vi "_visitCompoundGraphic.vi"(8 "error in (no error)":errorcluster, 10 "CompoundShape":refnum<class "CompoundShape.lvclass">, 11 "XMLExportVisitor in":refnum<class "XMLExportVisitor.lvclass">) -> (0 "error out":errorcluster, 2 "String":string, 3 "XMLExportVisitor out":refnum<class "XMLExportVisitor.lvclass">)   [LabVIEW 2018, in "XMLExportVisitor.lvclass"]
uses:
  XMLExportVisitor.lvclass
  C:/Users/fflores/Documents/LabVIEW-Open-Projects/LabIVEW OOP Design Patterns/Visitor Pattern/Visitor Class/Visitor.lvclass
  CompoundShape Class/CompoundShape.lvclass
  CompoundShape Class/CompoundShape.lvclass/CompoundShape.ctl
  Shape Class/Shape.lvclass
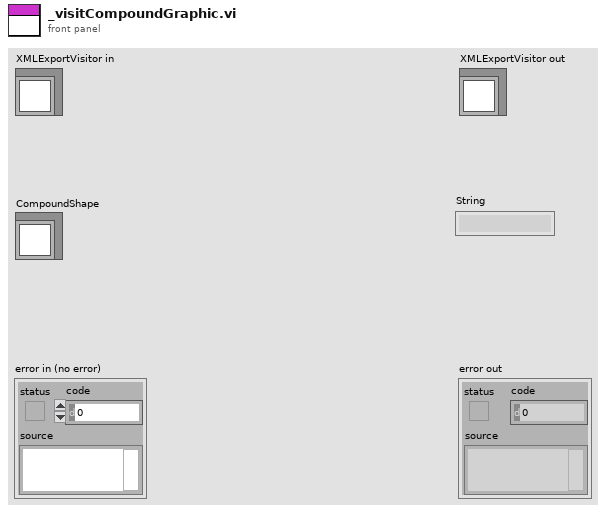
[diagram p1: front panel]
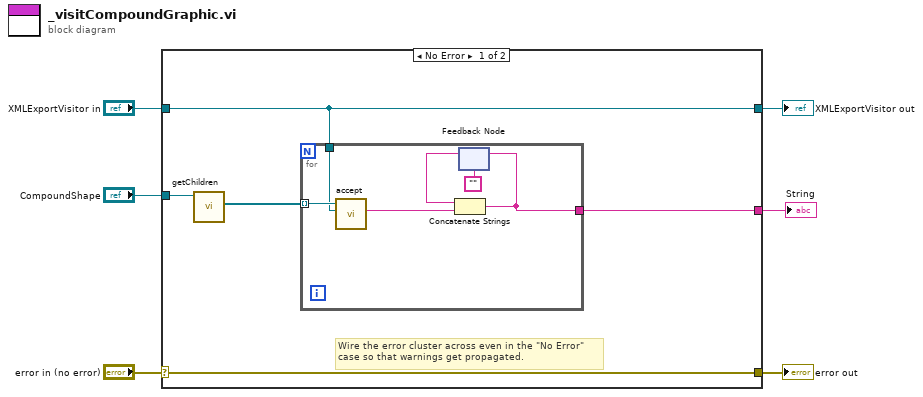
[diagram p0: block diagram]
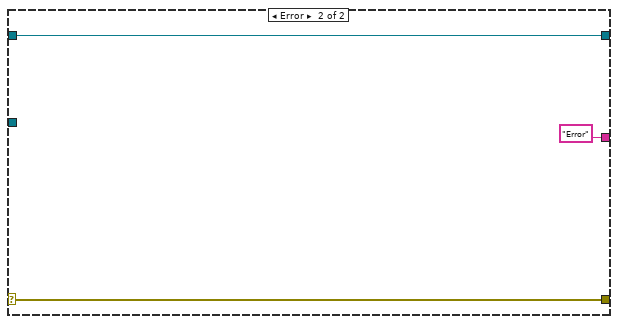
[diagram p2: hidden frame]
diagram:
  n1 = case shown="No Error" "error in (no error)" {
    selector: "error in (no error)" -> [w11 w20]
    tunnel: [w11 w20] -> w5
    tunnel: [w8 w19] -> w3
    tunnel: "XMLExportVisitor in" -> [w8 w19]
    tunnel: "CompoundShape" -> [w10 _]
    tunnel: [w9 "Error"] -> w1
    frame No Error {
      # "Wire the error cluster across even in the \"No Error\"\ncase so that warnings get propagated."
      n2 = call "getChildren.vi"("CompoundShape in"=w10) -> ("children"=w7:refnum<class "Shape.lvclass">[])  [unwired: 8 in, 2 out]
      n3 = for {
        tunnel: w7 -> [w17] mode=indexing
        tunnel: [w13] -> w9
        tunnel: w8 -> [w12]
        n4 = call-dynamic "accept.vi"("Visitor"=w12, "Shape in"=w17) -> ("String"=w16:string)  [unwired: 7 in, 2 out]
        n5 = feedback #1("") -> (w15:string)
        n6 = Concatenate Strings(w15, w16) -> (w13:string)
        n7 = feedback-in #1(w13) -> ()
      }
    }
    frame Error {
    }
  }
  "error out" <- w5
  "XMLExportVisitor out" <- w3
  "String" <- w1
